vi "Calibrate.vi"(8 "error in (no error)":errorcluster, 11 "KUKA youBot gripper motor in":refnum<class "NI_Robotics_KUKA youBot Gripper Motor_EtherCAT.lvclass">) -> (0 "error out":errorcluster, 3 "KUKA youBot gripper motor out":refnum<class "NI_Robotics_KUKA youBot Gripper Motor_EtherCAT.lvclass">)   [LabVIEW 2017, in "NI_Robotics_KUKA youBot Host.lvlib" / "NI_Robotics_KUKA youBot Gripper Motor_EtherCAT.lvclass"]
uses:
  <vilib>/robotics/KUKA youBot/Motor/Gripper Motor EtherCAT/NI_Robotics_KUKA youBot Gripper Motor_EtherCAT.lvclass
  c:/Program Files (x86)/National Instruments/LabVIEW 2017/vi.lib/robotics/KUKA youBot/Motor/Gripper Motor/NI_Robotics_KUKA youBot Gripper Motor.lvclass
  <vilib>/robotics/KUKA youBot/Motor/Gripper Motor EtherCAT/NI_Robotics_KUKA youBot Gripper Motor_EtherCAT.lvclass/NI_Robotics_KUKA youBot Gripper Motor_EtherCAT.ctl
  <vilib>/robotics/KUKA youBot/EtherCAT/EtherCAT Command.ctl
  <vilib>/robotics/KUKA youBot/EtherCAT/CmdCtrls/Param Cmd.ctl
  <vilib>/Platform/TimedLoop/XDataNode/timing_clust.ctl
  <vilib>/Platform/TimedLoop/XDataNode/nitl_modes.ctl
  <vilib>/Platform/TimedLoop/XDataNode/wakeup.ctl
  <vilib>/Platform/TimedLoop/XDataNode/XDataNode.xnode
  <vilib>/Platform/TimedLoop/XDataNode/XDNodeRunTimeDep.lvlib
  <vilib>/robotics/KUKA youBot/NI_Robotics_KUKA youBot Host.lvlib
  <vilib>/robotics/KUKA youBot/Motor/Gripper Motor/NI_Robotics_KUKA youBot Gripper Motor.lvclass
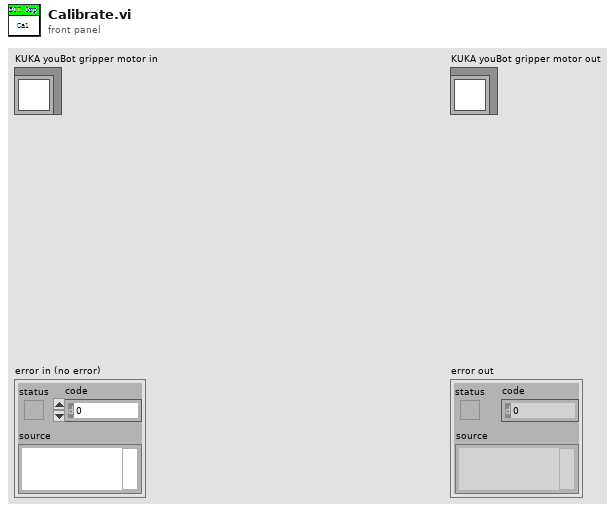
[diagram p1: front panel]
types:
  T1 = typedef "NI_Robotics_KUKA youBot Host.lvlib/EtherCAT Command.ctl" = cluster{"Module":u8, "Cmd":T2, "Type":u8, "Bank":u8, "Val":u32}
  T2 = typedef "NI_Robotics_KUKA youBot Host.lvlib/Param Cmd.ctl" = u8
  T3 = typedef "XDNodeRunTimeDep.lvlib/timing_clust.ctl" = cluster{"Expected End [f-1]":u64, "Actual End [f-1]":u64, "Finished Late? [f-1]":bool, "Expected End [i-1]":u64, "Actual End [i-1]":u64, "Finished Late? [i-1]":bool, "Expected Start [i]":u64, "Actual Start [i]":u64, "Expected Start [f]":u64, "Actual Start [f]":u64, "Source Name":string, "Structure Name":string, "Period":i64, "Deadline":i64, "Offset":i64, "Start":i64, "Priority":i32, "Timeout":i32, "Mode":T4, "Wakeup Reason":T5, "Error":errorcluster, "Source Type":string, "Secondary Source Type":string, "Global End Time":u64, "Global Start Time":u64, "Frame Duration":u64, "Iteration Duration":u64, "Assigned CPU":i32, "I/O Scan Engine Mode":u32}
  T4 = typedef "XDNodeRunTimeDep.lvlib/nitl_modes.ctl" = enum32{"No Change", "Process missed periods, maintain original phase", "Discard missed periods, maintain original phase", "Process missed periods, ignore original phase", "Discard missed periods, ignore original phase"}
  T5 = typedef "XDNodeRunTimeDep.lvlib/wakeup.ctl" = enum32{"Normal", "Aborted", "Asynchronous wakeup", "Timing source error", "Timed loop error", "Timeout"}
  T6 = typedef "NI_Robotics_KUKA youBot Host.lvlib/Mater Handler.ctl" = i32
  T7 = typedef "NI_Robotics_KUKA youBot Host.lvlib/EtherCAT Reply.ctl" = cluster{"replyAddr":u8, "moduleAddr":u8, "status":u8, "Cmd":u8, "Val":i32}
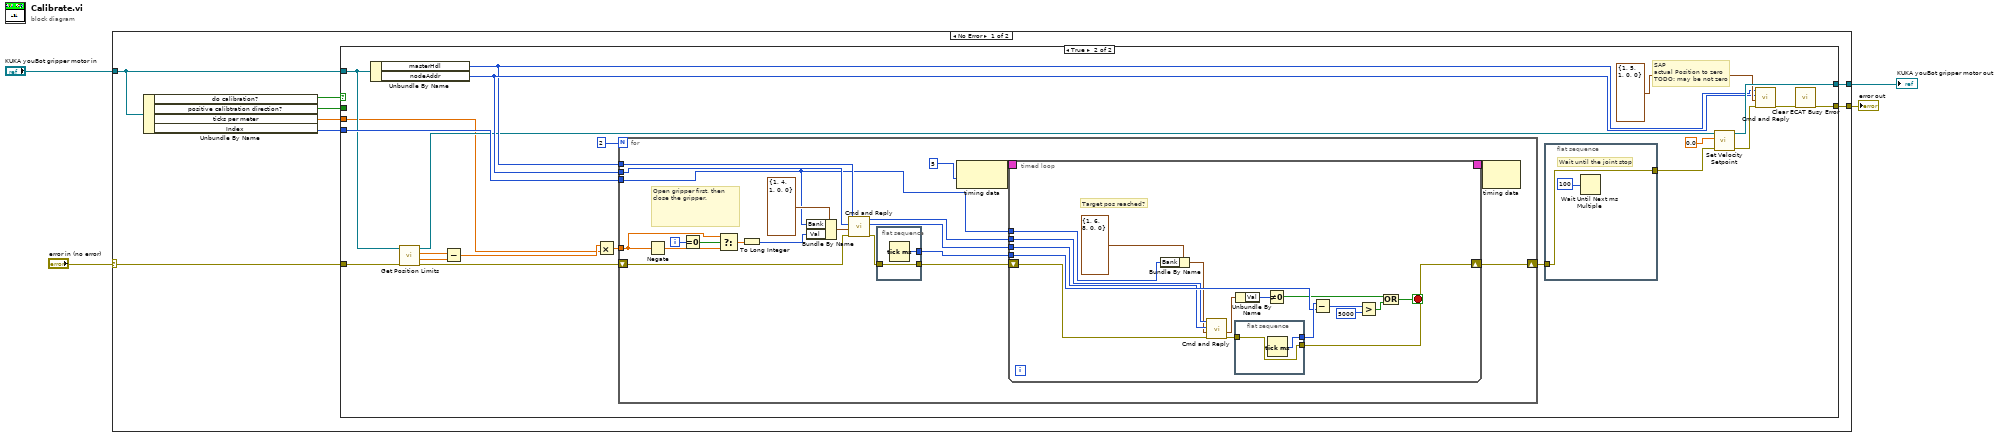
[diagram p0: block diagram]
diagram:
  n1 = case shown="No Error" "error in (no error)" {
    selector: "error in (no error)" -> [w6 w87]
    tunnel: "KUKA youBot gripper motor in" -> [w11 w86]
    tunnel: [w8 w86] -> w2
    tunnel: [w7 w87] -> w1
    frame No Error {
      n2 = Unbundle By Name(w11) -> ("do calibration?"=w12:bool, "positive calibtration direction?"=w10:bool, "ticks per meter"=w9:dbl, "Index"=w5:i32)
      n3 = case shown="True" w12 {
        tunnel: w11 -> [w14 w21]
        tunnel: w10 -> [_ _]
        tunnel: w9 -> [_ w15]
        tunnel: [w14 w32] -> w8
        tunnel: [w13 w16] -> w7
        tunnel: w6 -> [w13 w30]
        tunnel: w5 -> [_ w22]
        frame False {
        }
        frame True {
          # "SAP\nactual Position to zero\nTODO: may be not zero"
          n4 = Unbundle By Name(w21) -> ("masterHdl"=w19:T6, "nodeAddr"=w20:u16)
          n5 = call <vilib>:"Get Position Limits.vi"("error in (no error)"=w30, "KUKA youBot gripper motor in"=w21) -> ("error out"=w25:errorcluster, "min dist (m)"=w28:dbl, "max dist (m)"=w29:dbl, "KUKA youBot gripper motor out"=w18:refnum<class "NI_Robotics_KUKA youBot Gripper Motor_EtherCAT.lvclass">)  [unwired: 6 in]
          n6 = Subtract(x=w29, y=w28) -> (x-y=w27:dbl)
          n7 = Multiply(x=w27, y=w15) -> (x*y=w26:dbl)
          n8 = for {
            N: 2 -> [_]
            tunnel: w26 -> [w36]
            shift-right: [w53] -> w35
            shift-left: w25 -> [w52]
            tunnel: w22 -> [w39]
            tunnel: w20 -> [w48]
            tunnel: w19 -> [w47]
            i -> [w50]
            # "Open gripper first, then close the gripper."
            n9 = Negate(x=w36) -> (-x=w37:dbl)
            n10 = Equal To 0?(x=w50) -> (x = 0?=w49:bool)
            n11 = Select(t=w36, s=w49, f=w37) -> (s? t:f=w43:dbl)
            n12 = To Long Integer(number=w43) -> (32bit integer=w42:i32)
            n13 = Bundle By Name(cluster=T1 {"Module"=1, "Cmd"=4, "Type"=1, "Bank"=0, "Val"=0} ("EtherCAT Command"), "Bank"=w39, "Val"=w42) -> (w45:T1)
            n14 = call <vilib>:"Cmd and Reply.vi"("error in (no error)"=w52, "EtherCAT command"=w45, "nodeAddr in"=w48, "masterHdl in"=w47) -> ("error out"=w51:errorcluster, "nodeAddr out"=w46:u16, "masterHdl out"=w41:T6)  [unwired: 3 in, 2 out]
            n15 = flat-sequence {
              tunnel: [w58] -> w54
              tunnel: [w57] -> w40
              tunnel: w51 -> [w57]
              frame #0 {
                n16 = Tick Count (ms)() -> (millisecond timer value=w58:u32)
              }
            }
            n17 = node-c288(i64 5 ("Period")) -> (w56:T3)
            n18 = timed-loop {
              timing: w56 -> [_]
              timing-out: [_] -> w55
              shift-right: [w74] -> w53
              shift-left: w40 -> [w68]
              tunnel: w54 -> [w72]
              tunnel: w41 -> [w67]
              tunnel: w46 -> [w66]
              tunnel: w39 -> [w60]
              stop <- w75 stop-if-true
              # "Target pos reached?"
              n19 = Bundle By Name(cluster=T1 {"Module"=1, "Cmd"=6, "Type"=8, "Bank"=0, "Val"=0} ("EtherCAT Command"), "Bank"=w60) -> (w61:T1)
              n20 = call <vilib>:"Cmd and Reply.vi"("error in (no error)"=w68, "EtherCAT command"=w61, "nodeAddr in"=w66, "masterHdl in"=w67) -> ("error out"=w59:errorcluster, "EtherCAT reply"=w65:T7)  [unwired: 3 in, 3 out]
              n21 = flat-sequence {
                tunnel: w59 -> [w77]
                tunnel: [w77] -> w74
                tunnel: [w76] -> w73
                frame #0 {
                  n22 = Tick Count (ms)() -> (millisecond timer value=w76:u32)
                }
              }
              n23 = Unbundle By Name(w65) -> ("Val"=w63:i32)
              n24 = Not Equal To 0?(x=w63) -> (x != 0?=w64:bool)
              n25 = Subtract(x=w73, y=w72) -> (x-y=w71:u32)
              n26 = Greater?(x=w71, y=u32 5000) -> (0:w69:bool)
              n27 = Compound Arithmetic op=OR(w64, w69) -> (w75:bool)
            }
            n28 = node-c288(w55) -> ()  [unwired: 1 out]
          }
          n29 = flat-sequence {
            tunnel: w35 -> [w84]
            tunnel: [w84] -> w24
            frame #0 {
              # "Wait until the joint stop"
              n30 = Wait Until Next ms Multiple(millisecond multiple=u32 100) -> ()  [unwired: 1 out]
            }
          }
          n31 = call-dynamic "Set Velocity Setpoint.vi"("error in (no error)"=w24, "ccw velocity (rpm)"=0.0, "KUKA youBot gripper motor in"=w18) -> ("error out"=w33:errorcluster, "KUKA youBot gripper motor out"=w32:refnum<class "NI_Robotics_KUKA youBot Gripper Motor_EtherCAT.lvclass">)  [unwired: 7 in]
          n32 = call <vilib>:"Cmd and Reply.vi"("error in (no error)"=w33, "EtherCAT command"=T1 {"Module"=1, "Cmd"=5, "Type"=1, "Bank"=0, "Val"=0} ("EtherCAT Command"), "nodeAddr in"=w20, "masterHdl in"=w19) -> ("error out"=w17:errorcluster)  [unwired: 3 in, 4 out]
          n33 = call <vilib>:"Clear ECAT Busy Error.vi"("error in (no error)"=w17) -> ("error out"=w16:errorcluster)  [unwired: 10 in]
        }
      }
    }
    frame Error {
    }
  }
  "error out" <- w1
  "KUKA youBot gripper motor out" <- w2
